vi "CheckAllSignalsInSameFrame.vi"(8 "error in":errorcluster, 10 "Input Channel Selections":T1[](array[typedef]) {"Data Type" items=["Signed", "Unsigned", "IEEE Float"]}, 11 "Rolling Counter and CRC":T1[](array[typedef]) {"Data Type" items=["Signed", "Unsigned", "IEEE Float"]}) -> (0 "error out":errorcluster, 3 "Pass?":bool)   [LabVIEW 2016, in "LIN Frame Protection Addon System Explorer.lvlib"]
uses:
  LIN Frame Protection Addon System Explorer.lvlib
  Shared/Types/InputChannelConfiguration.ctl
  Shared/LIN Frame Protection Addon Shared.lvlib
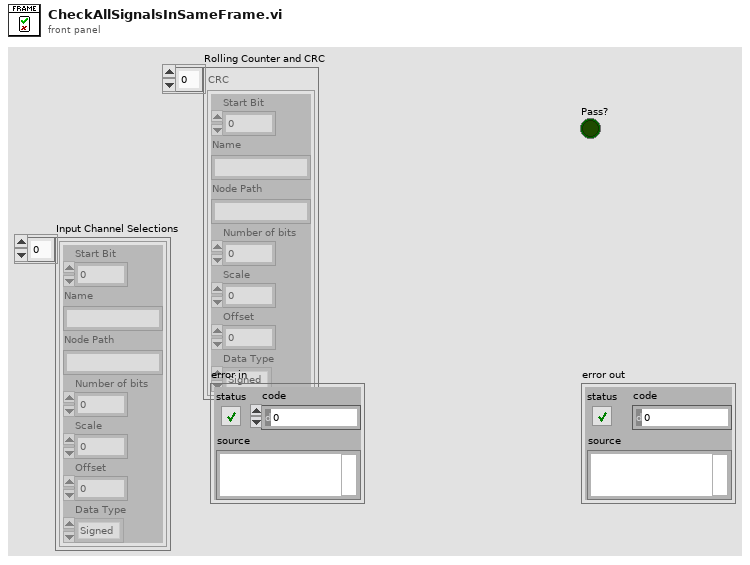
[diagram p1: front panel]
types:
  T1 = typedef "LIN Frame Protection Addon Shared.lvlib/InputChannelConfiguration.ctl" = cluster{"Start Bit":i32, "Name":string, "Node Path":string, "Number of bits":i32, "Scale":dbl, "Offset":dbl, "Data Type":u32}
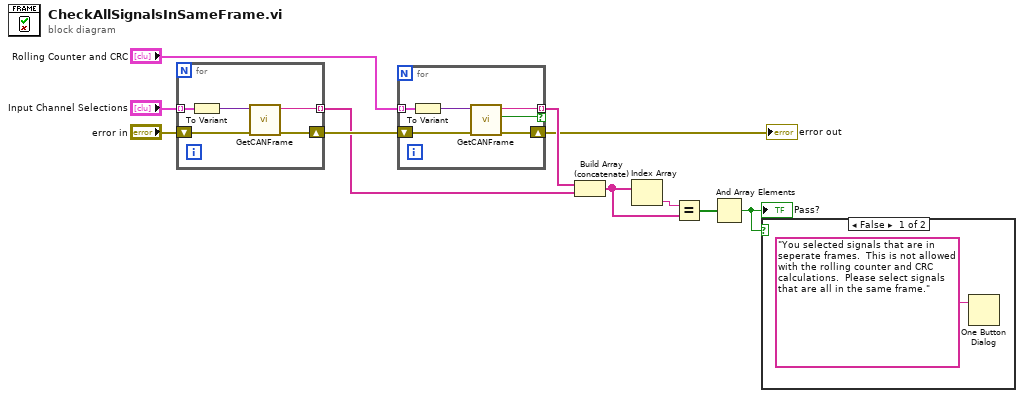
[diagram p0: block diagram]
diagram:
  n1 = for {
    tunnel: [w16] -> w6 mode=indexing
    tunnel: "Input Channel Selections" -> [w15] mode=indexing
    shift-right: [w13] -> w10
    shift-left: "error in" -> [w12]
    n2 = To Variant(anything=w15) -> (Variant=w14:variant)
    n3 = call "GetCANFrame.vi"("error in (no error)"=w12, "Variant"=w14) -> ("error out"=w13:errorcluster, "PathArrayToString"=w16:string)  [unwired: 7 in, 1 out]
  }
  n4 = for {
    tunnel: [w22] -> w7 mode=indexing if=w17
    tunnel: "Rolling Counter and CRC" -> [w21] mode=indexing
    shift-right: [w19] -> w2
    shift-left: w10 -> [w18]
    n5 = To Variant(anything=w21) -> (Variant=w20:variant)
    n6 = call "GetCANFrame.vi"("error in (no error)"=w18, "Variant"=w20) -> ("error out"=w19:errorcluster, "Valid?"=w17:bool, "PathArrayToString"=w22:string)  [unwired: 7 in]
  }
  "error out" <- w2
  n7 = Build Array (concatenate)(w7, w6) -> (w4:string[])
  n8 = Index Array(array=w4) -> (element=w5:string)  [unwired: 1 in]
  n9 = Equal?(x=w5, y=w4) -> (x = y?=w3:bool[])
  n10 = And Array Elements(Boolean array=w3) -> (logical AND=w1:bool)
  "Pass?" <- w1
  n11 = case shown="False" w1 {
    frame False {
      n12 = One Button Dialog(message="You selected signals that are in seperate frames.  This is not allowed with the rolling counter and CRC calculations.  Please select signals that are all in the same frame.") -> ()  [unwired: 1 in, 1 out]
    }
    frame True {
    }
  }
